vi "Accept Or Decline.vi"(6 "Additional Events":T1, 7 "timeout":i32=200, 8 "error in (no error)":errorcluster, 9 "AutoAccept":bool, 10 "MM Gui Updates In":refnum<queue>, 11 "MM Button Events In":refnum<notifier>) -> (0 "error out":errorcluster, 1 "Accepted or Declined":T2, 2 "MM Gui Updates Out":refnum<queue>, 3 "Button Events Out":refnum<notifier>)   [LabVIEW 2009]
uses:
  MixedMode/Messages/Mixed Mode Button Events Message.ctl
  MixedMode/Messages/Mixed Mode Button Events.ctl
  Mixed Mode Widget Button States.ctl
  MixedMode/Messages/Mixed Mode Gui Update Msg.ctl
  MixedMode/Messages/Mixed Mode GUI Update Type.ctl
  MixedMode/Messages/Target.ctl
  Data Access Objects/Metadata/LBCB Number.ctl
  Accepted or Declined.ctl
  Monitor Button Events.ctl
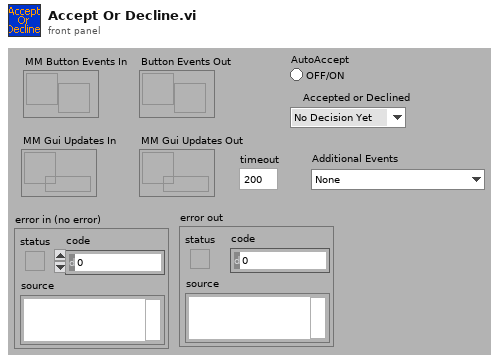
[diagram p1: front panel]
types:
  T1 = typedef "Monitor Button Events.ctl" = enum16{"None", "Running Event", "Connect NTCP Server Event"}
  T2 = typedef "Accepted or Declined.ctl" = enum16{"No Decision Yet", "Accepted", "Declined", "Abort"}
  T3 = typedef "Mixed Mode Gui Update Msg.ctl" = cluster{"MM GUI Update Type":T4, "Targets":T5[], "State":bool, "Step":string}
  T4 = typedef "Mixed Mode GUI Update Type.ctl" = enum16{"Nop", "Targets", "Accept.Blink", "Start.Blink", "TestStats", "Control.Enabled", "StartTestTimer", "RunInputFile", "NTCP Server", "Propose.Auto", "Execute.Auto"}
  T5 = typedef "Target.ctl" = cluster{"LBCB Number":T6, "DOF Vectors":enum16{" ", "Dx", "Dy", "Dz", "Rx", "Ry", "Rz", "Fx", "Fy", "Fz", "Mx", "My", "Mz"}, "Amount":dbl}
  T6 = typedef "LBCB Number.ctl" = enum16{"LBCB1", "LBCB2"}
  T7 = typedef "Mixed Mode Button Events Message.ctl" = cluster{"MM Control Events":T8, "Button States":T9}
  T8 = typedef "Mixed Mode Button Events.ctl" = enum16{"Propose.Accept", "Propose.Decline", "Execute.Start", "Execute.Stop", "TargetSet", "InputFile.Load", "InputFile.Reset", "InputFile.Pause", "InputFile.Run", "CartesianType.Changed", "NCTP.ConnectToServer", "NTCP.DisconnectFromServer", "Application.Stop", "Control.Enabled", "Control.Disabled", "ControlType.Changed", "Nop"}
  T9 = typedef "Mixed Mode Widget Button States.ctl" = cluster{"Auto-Start Enabled":bool, "Auto-Accept Enabled":bool, "Exit Requested":bool, "Input File Loaded":bool, "Input File Running":bool, "NTCP Server  On":bool}
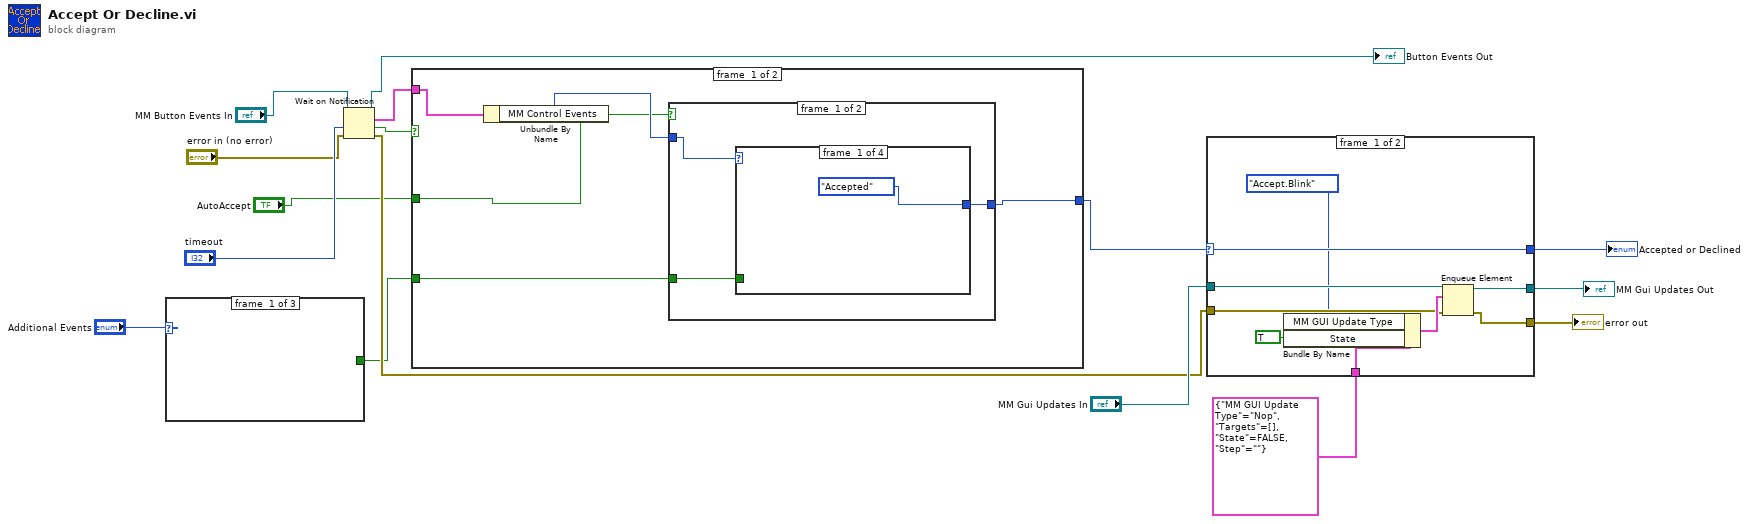
[diagram p0: block diagram]
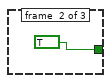
[diagram p2: hidden frame]
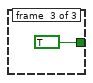
[diagram p3: hidden frame]
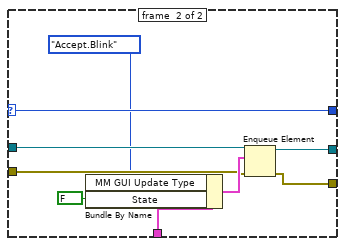
[diagram p4: hidden frame]
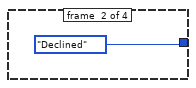
[diagram p5: hidden frame]
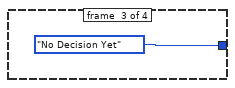
[diagram p6: hidden frame]
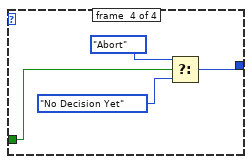
[diagram p7: hidden frame]
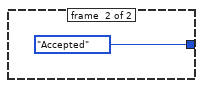
[diagram p8: hidden frame]
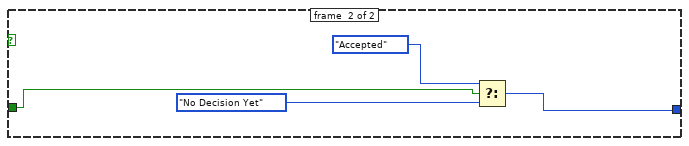
[diagram p9: hidden frame]
diagram:
  n1 = case shown="\"Connect NTCP Server Event\"" "Additional Events" {
    tunnel: [_ TRUE TRUE] -> w2
    frame #0 {
    }
    frame #1 {
    }
    frame #2 {
    }
  }
  n2 = Wait on Notification(notifier="MM Button Events In", timeout in ms (-1)="timeout", error in (no error)="error in (no error)") -> (notifier out=→"Button Events Out":refnum<notifier>, notification=w11:T7, timed out?=w12:bool, error out=w4:errorcluster)  [unwired: 1 in]
  n3 = case shown="False" w12 {
    tunnel: w11 -> [w23 _]
    tunnel: [w21 w37] -> w10
    tunnel: w2 -> [w20 _]
    tunnel: "AutoAccept" -> [w19 w36]
    frame #0 {
      n4 = Unbundle By Name(w23) -> ("MM Control Events"=w22:T8)
      n5 = case shown="False" w19 {
        tunnel: w22 -> [w26 _]
        tunnel: [w25 Accepted_or_Declined."Accepted" ("Accepted or Declined")] -> w21
        tunnel: w20 -> [w24 _]
        frame #0 {
          n6 = case shown="\"NTCP.DisconnectFromServer\"" w26 {
            tunnel: [Accepted_or_Declined."Accepted" ("Accepted or Declined") Accepted_or_Declined."Declined" ("Accepted or Declined") Accepted_or_Declined."No Decision Yet" ("Accepted or Declined") w31] -> w25
            tunnel: w24 -> [_ _ _ w33]
            frame #0 {
            }
            frame #1 {
            }
            frame #2 {
            }
            frame #3 {
              n7 = Select(t=Accepted_or_Declined."Abort", s=w33, f=Accepted_or_Declined."No Decision Yet" ("Accepted or Declined")) -> (s? t:f=w31:T2)
            }
          }
        }
        frame #1 {
        }
      }
    }
    frame #1 {
      n8 = Select(t=Accepted_or_Declined."Accepted", s=w36, f=Accepted_or_Declined."No Decision Yet" ("Accepted or Declined")) -> (s? t:f=w37:T2)
    }
  }
  n9 = case shown="\"Accepted\", Default" w10 {
    selector: w10 -> [w47 w56]
    tunnel: [w47 w56] -> w9
    tunnel: "MM Gui Updates In" -> [w46 w55]
    tunnel: T3 {"MM GUI Update Type"=enum."Nop", "Targets"=[], "State"=FALSE, "Step"=""} ("element") -> [w45 w54]
    tunnel: [w43 w52] -> w6
    tunnel: [w42 w51] -> w5
    tunnel: w4 -> [w41 w50]
    frame #0 {
      n10 = Bundle By Name(cluster=w45, "MM GUI Update Type"=Mixed_Mode_GUI_Update_Type."Accept.Blink", "State"=TRUE) -> (w44:T3)
      n11 = Enqueue Element(queue=w46, element=w44, error in (no error)=w41) -> (queue out=w43:refnum<queue>, error out=w42:errorcluster)  [unwired: 1 in, 1 out]
    }
    frame #1 {
      n12 = Bundle By Name(cluster=w54, "MM GUI Update Type"=Mixed_Mode_GUI_Update_Type."Accept.Blink", "State"=FALSE) -> (w53:T3)
      n13 = Enqueue Element(queue=w55, element=w53, error in (no error)=w50) -> (queue out=w52:refnum<queue>, error out=w51:errorcluster)  [unwired: 1 in, 1 out]
    }
  }
  "Accepted or Declined" <- w9
  "MM Gui Updates Out" <- w6
  "error out" <- w5
